vi "send json with size.vi"(6 "addr/port":cluster{"address":string, "port":i32}={"address"="127.0.0.1", "port"=31415}, 8 "error in":errorcluster, 11 "json string":string) -> (0 "error out":errorcluster, 2 "bytes written":i32, 3 "connection ID out":refnum<k5>)   [LabVIEW 2015]
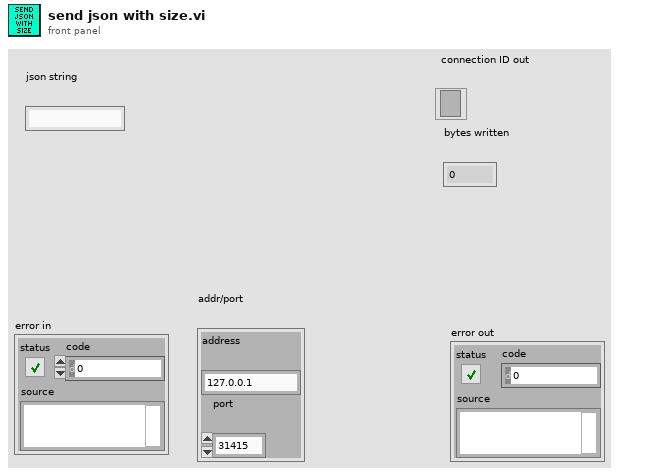
[diagram p1: front panel]
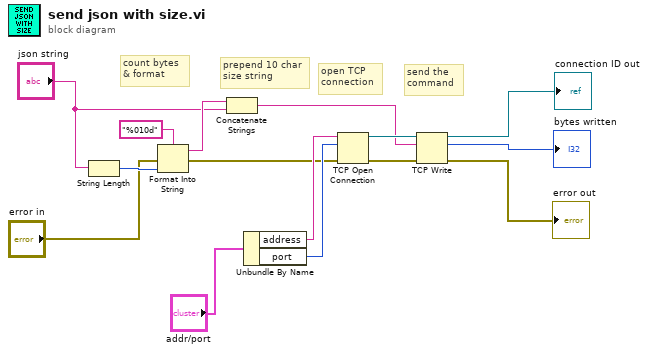
[diagram p0: block diagram]
diagram:
  # "prepend 10 char\nsize string"
  # "count bytes \n& format"
  # "send the \ncommand"
  # "open TCP\nconnection"
  n1 = String Length(string="json string") -> (length=w7:i32)
  n2 = Format Into String(format string="%010d", error in="error in", w7) -> (resulting string=w3:string, error out=w4:errorcluster)  [unwired: 1 in]
  n3 = Concatenate Strings(w3, "json string") -> (w5:string)
  n4 = Unbundle By Name("addr/port") -> ("address"=w11:string, "port"=w12:i32)
  n5 = TCP Open Connection(address=w11, remote port or service name=w12, error in (no error)=w4) -> (connection ID=w15:refnum<k5>, error out=w14:errorcluster)  [unwired: 2 in]
  n6 = TCP Write(connection ID=w15, data in=w5, error in (no error)=w14) -> (connection ID out=→"connection ID out":refnum<k5>, bytes written=→"bytes written":i32, error out=→"error out":errorcluster)  [unwired: 1 in]
